vi "convert to 8bits.vi"(9 "max":dbl, 10 "min":dbl, 11 "input":dbl) -> (3 "output_8b":dbl)   [LabVIEW 2014]
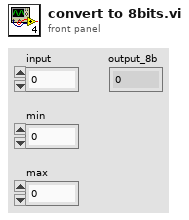
[diagram p1: front panel]
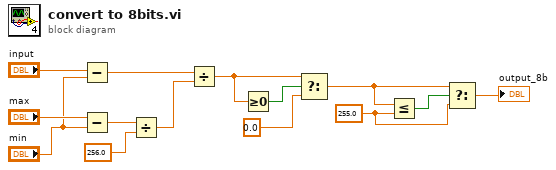
[diagram p0: block diagram]
diagram:
  w2 = 255.0 ("y")
  n1 = Subtract(x="input", y="min") -> (x-y=w9:dbl)
  n2 = Subtract(x="max", y="min") -> (x-y=w13:dbl)
  n3 = Divide(x=w13, y=256.0) -> (x/y=w8:dbl)
  n4 = Divide(x=w9, y=w8) -> (x/y=w6:dbl)
  n5 = Greater Or Equal To 0?(x=w6) -> (x >= 0?=w7:bool)
  n6 = Select(t=w6, s=w7, f=0.0) -> (s? t:f=w3:dbl)
  n7 = Less Or Equal?(x=w3, y=w2) -> (x <= y?=w4:bool)
  n8 = Select(t=w3, s=w4, f=w2) -> (s? t:f=→"output_8b":dbl)
